vi "Open Connection_ni9485.vi"(8 "error in (no error)":errorcluster, 9 "ni9485":T1={"crio_interlock[72]"=[FALSE, FALSE, FALSE, FALSE, FALSE, FALSE, FALSE, FALSE, FALSE, FALSE, FALSE, FALSE, FALSE, FALSE, FALSE, FALSE, FALSE, FALSE, FALSE, FALSE, FALSE, FALSE, FALSE, FALSE, FALSE, FALSE, FALSE, FALSE, FALSE, FALSE, FALSE, FALSE, FALSE, FALSE, FALSE, FALSE, FALSE, FALSE, FALSE, FALSE, FALSE, FALSE, FALSE, FALSE, FALSE, FALSE, FALSE, FALSE, FALSE, FALSE, FALSE, FALSE, FALSE, FALSE, FALSE, FALSE, FALSE, FALSE, FALSE, FALSE, FALSE, FALSE, FALSE, FALSE, FALSE, FALSE, FALSE, FALSE, FALSE, FALSE, FALSE, FALSE]}, 10 "topicName":string) -> (0 "error out":errorcluster, 3 "topicRef":cluster{"topicName":string, "type":refnum<vi>})   [LabVIEW 2015]
uses:
  SALTypedefs/m2ms/ni9485.ctl
  SALTypedefs/m2ms/m2ms.lvlib
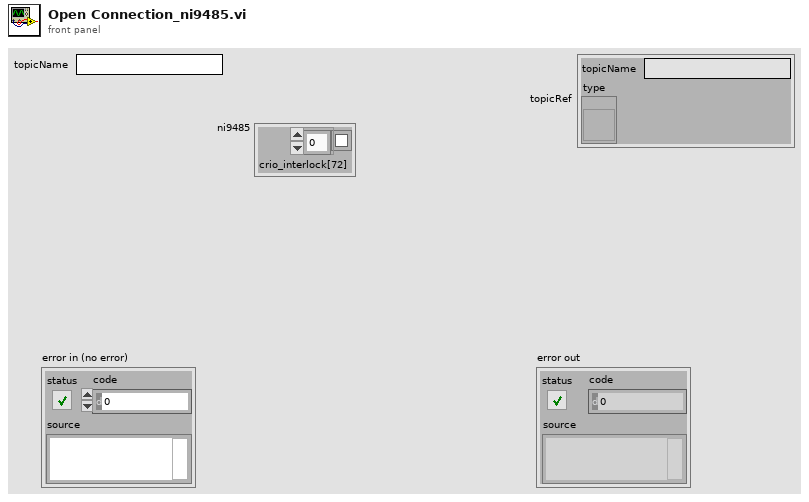
[diagram p1: front panel]
types:
  T1 = typedef "m2ms.lvlib/ni9485.ctl" = cluster{"crio_interlock[72]":bool[]}
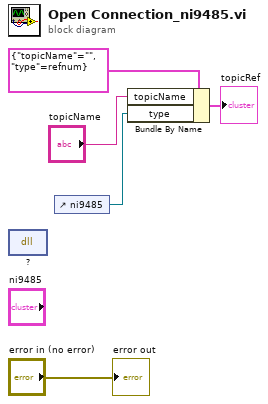
[diagram p0: block diagram]
diagram:
  n1 = dll-call lib="?" fn="?"() -> ()  [unwired: 4 in, 2 out]
  n2 = control-ref of="ni9485"() -> (w2:refnum<vi>)
  n3 = Bundle By Name(cluster=cluster{"topicName":string, "type":refnum<vi>} {"topicName"="", "type"=refnum} ("topicRef"), "topicName"="topicName", "type"=w2) -> (→"topicRef":cluster{"topicName":string, "type":refnum<vi>})
  "error out" <- "error in (no error)"
